vi "设置布尔控件值.vi"(1 "布尔":bool, 2 "error in (no error)":errorcluster caption="错误输入（无错误）", 3 "布尔控件":refnum<vi>) -> (0 "error out":errorcluster caption="错误输出")   [LabVIEW 2014]
doc: "该模板用于创建子VI。"
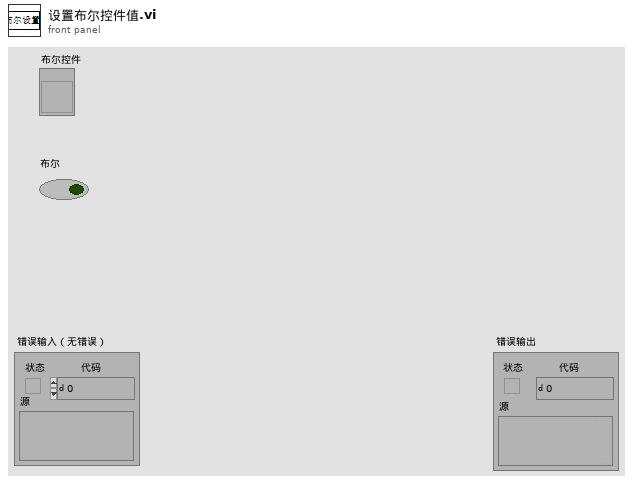
[diagram p1: front panel]
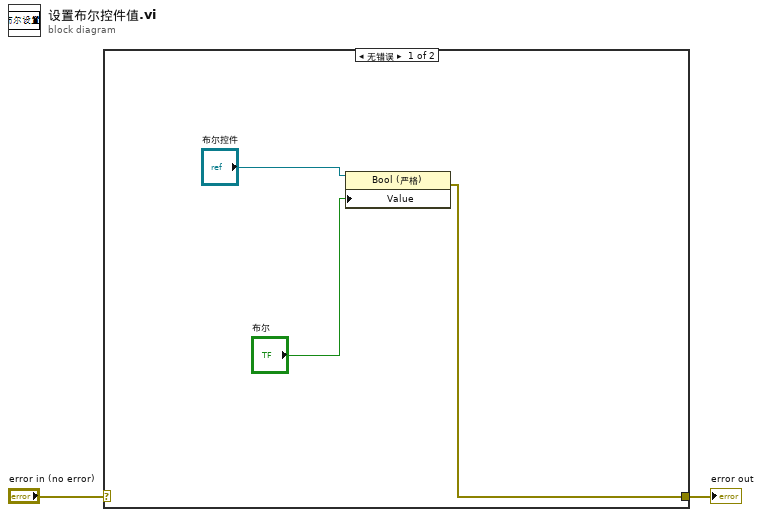
[diagram p0: block diagram]
diagram:
  n1 = case shown="无错误" "error in (no error)" {
    selector: "error in (no error)" -> [_ w6]
    tunnel: [w3 w6] -> w1
    frame No Error {
      n2 = property class="Bool (严格)"(reference="布尔控件", "Value"="布尔") -> (error out=w3:errorcluster)  [unwired: 1 in, 1 out]
    }
    frame Error {
    }
  }
  "error out" <- w1
